vi "initAcq.vi"(7 "Session":path=path "Z:/users/Manolis/Labview/Water Conditioning/sessions_Win7.dsn", 8 "error in (no error)":errorcluster, 9 "password":string="manolis#1", 10 "userID":string="manolis", 11 "Acquisition in":refnum<class "Acquisition.lvclass">) -> (0 "error out":errorcluster, 3 "Acquisition out":refnum<class "Acquisition.lvclass">)   [LabVIEW 2014, in "Acquisition.lvclass"]
uses:
  Acquisition.lvclass
  Scanner/Database/Database.lvclass
  Acquisition.lvclass/Acquisition.ctl
panel:
  in  "Cluster":T1
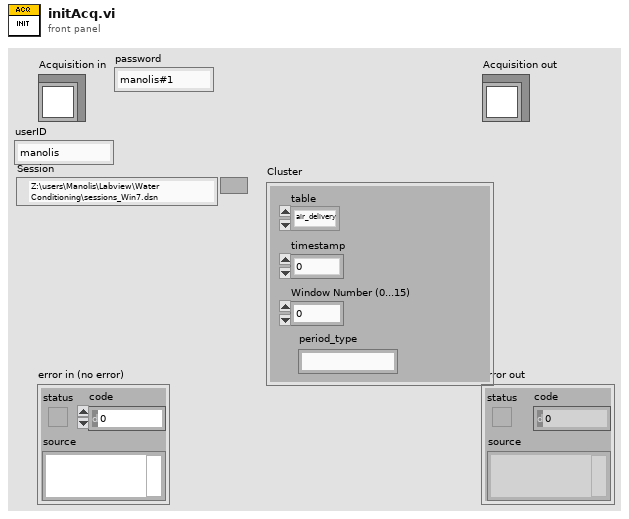
[diagram p1: front panel]
types:
  T1 = cluster{"table":enum16{"air_delivery", "beh_session", "stim_periods", "licks", "liquid_delivery"}, "timestamp":dbl, "Window Number (0...15)":i32, "period_type":string}
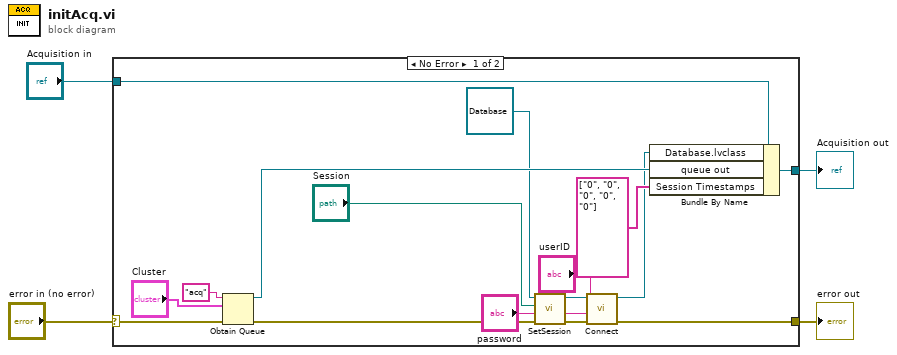
[diagram p0: block diagram]
diagram:
  n1 = case shown="No Error" "error in (no error)" {
    selector: "error in (no error)" -> [w17 w22]
    tunnel: [w7 w22] -> w3
    tunnel: [w19 w21] -> w1
    tunnel: "Acquisition in" -> [w20 w21]
    frame No Error {
      n2 = Obtain Queue(name (unnamed)="acq", element data type="Cluster", error in (no error)=w17) -> (queue out=w15:refnum<queue>, error out=w11:errorcluster)  [unwired: 2 in, 1 out]
      n3 = call-dynamic "SetSession.vi"("error in (no error)"=w11, "Session"="Session", "Database in"=refnum<class "Database.lvclass"> refnum ("Database.lvclass")) -> ("error out"=w8:errorcluster, "Database out"=w10:refnum<class "Database.lvclass">)  [unwired: 7 in]
      n4 = call-dynamic "Connect.vi"("Database in"=w10, "userID"="userID", "password"="password", "error in (no error)"=w8) -> ("Database out"=w9:refnum<class "Database.lvclass">, "error out"=w7:errorcluster)  [unwired: 5 in]
      n5 = Bundle By Name(cluster=w20, "Database.lvclass"=w9, "queue out"=w15, "Session Timestamps"=string[] ["0", "0", "0", "0", "0"]) -> (w19:refnum<class "Acquisition.lvclass">)
    }
    frame Error {
    }
  }
  "error out" <- w3
  "Acquisition out" <- w1
